vi "Test program 5.vi"() -> ()   [LabVIEW 2013, in "Keithly user program.lvlib"]
uses:
  Keithly user program.lvlib
  Typedefs/KE622x -- On Off Control.ctl
  Configure/Output/Typedefs/KE6221 -- Output Response.ctl
  Configure/Source/Typedefs/KE622x -- Current Range.ctl
  Configure/Source/Typedefs/KE622x -- Current Level.ctl
  Configure/Source/Typedefs/KE622x -- Voltage Limit.ctl
  Configure/Utility/Typedefs/KE622x -- Instrument Type.ctl
panel:
  in  "Current Level (A) 2":T1=0.1 min=-0.105 max=0.105 format="%.4p"
  in  "stop 2":bool
  in  "stop":bool
  out "XY Graph":cluster{"X":dbl, "Y":dbl}[](graph)
  in  "2182 -A Params In":T2={"Auto Range?"=FALSE, "Man / Selected\n       Range"=enum."10mV", "Enable Digital\n       Filter?"=FALSE, "Filter Type"=enum."Movin", "Filter Count"=1, "      Filter\nWindow (%)"=0.01, "Enable Analog\n       Filter?"=FALSE, "NPLCs"=5} {"NPLCs" min=1 max=10; "Filter\nWindow (%)" min=0.01 max=10.0 step=0.01 format="%.2f"; "Filter Count" min=1 max=100}
  in  "Voltage Limit (V)":T3=10.0 min=0.1 max=105.0 step=0.01 format="%.2p"
  in  "Current Level (A)":T1=0.1 min=-0.105 max=0.105 format="%.4p"
  in  "Current Range":T4
  in  "KE6221 Output Response":T5=enum."Slow"
  in  "Analog Filter State":T6
  in  "VISA resource name":refnum<visa-resource-name>
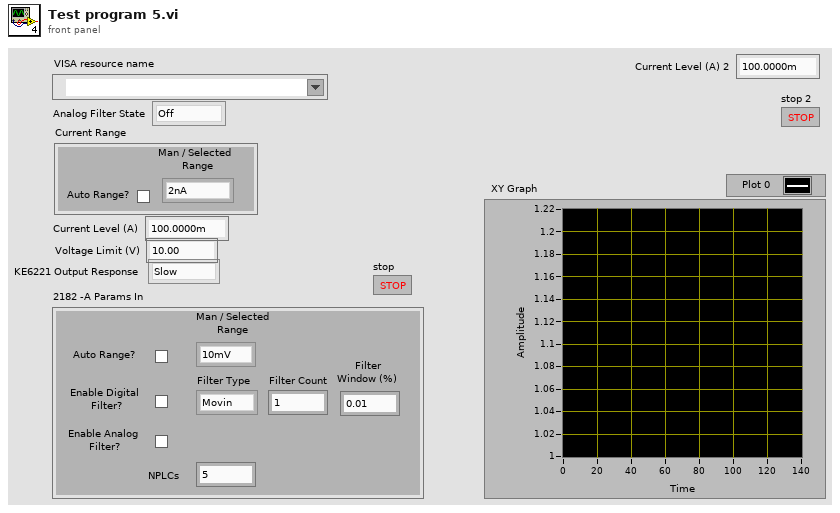
[diagram p1: front panel]
types:
  T1 = typedef "Keithly user program.lvlib/KE622x -- Current Level.ctl" = dbl
  T2 = cluster{"Auto Range?":bool, "Man / Selected\n       Range":enum16{"10mV", "100mV", "1V", "10V", "100V"}, "Enable Digital\n       Filter?":bool, "Filter Type":enum16{"Movin", "Repeat"}, "Filter Count":u32, "      Filter\nWindow (%)":dbl, "Enable Analog\n       Filter?":bool, "NPLCs":u32}
  T3 = typedef "Keithly user program.lvlib/KE622x -- Voltage Limit.ctl" = dbl
  T4 = typedef "Keithly user program.lvlib/KE622x -- Current Range.ctl" = cluster{"Auto Range?":bool, "Man / Selected\n        Range":enum16{"2nA", "20nA", "200nA", "2uA", "20uA", "200uA", "2mA", "20mA", "100mA"}}
  T5 = typedef "Keithly user program.lvlib/KE6221 -- Output Response.ctl" = enum16{"Fast", "Slow"}
  T6 = typedef "Keithly user program.lvlib/KE622x -- On Off Control.ctl" = enum16{"Off", "On"}
  T7 = typedef "Keithly user program.lvlib/KE622x -- Instrument Type.ctl" = enum16{"KE6220", "KE6221"}
  T8 = cluster{"Auto Range?":bool, "Man / Selected\n        Range":u16, "Enable Digital\n       Filter?":bool, "Filter Type":u16, "Filter Count":u32, "      Filter\nWindow (%)":dbl, "Enable Analog\n       Filter?":bool, "NPLCs":u32}
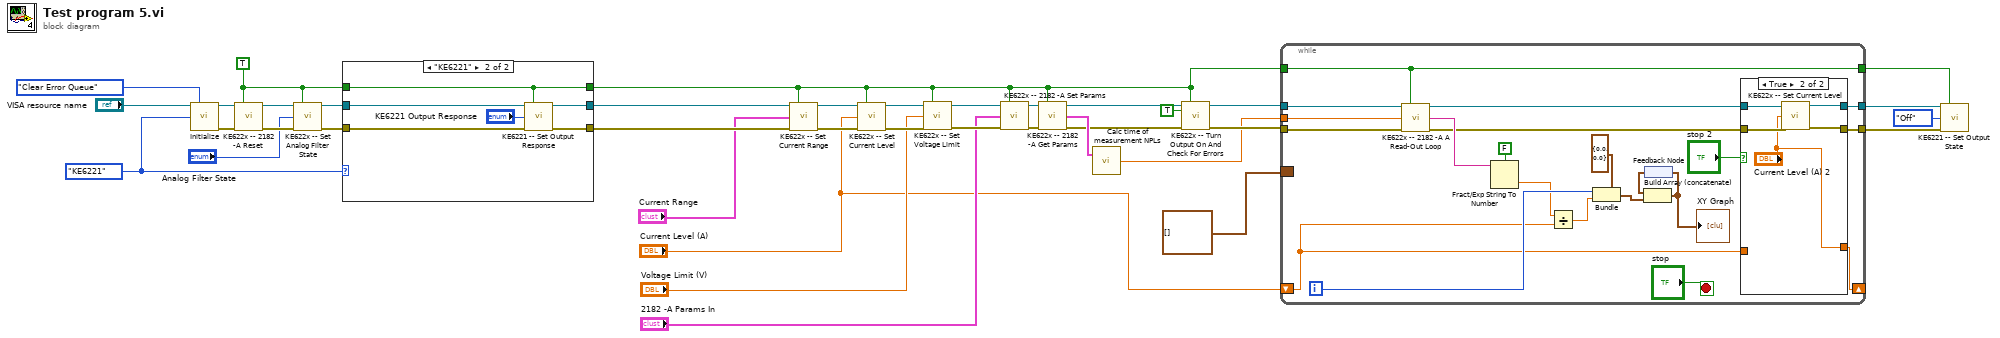
[diagram p0: block diagram]
diagram:
  w28 = TRUE ("Check For SCPI Errors? (T)")
  w29 = KE622x_--_Instrument_Type."KE6221" ("Instrument Type")
  n1 = call "Initialize.vi"("VISA resource name"="VISA resource name", "Error Queue Option"=enum16{"Clear Error Queue", "Error Query"}."Clear Error Queue", "Instrument Type"=w29) -> ("VISA resource name out"=w36:refnum<visa-resource-name>, "error out"=w35:errorcluster)  [unwired: 11 in]
  n2 = call "KE622x -- 2182 -A Reset.vi"("622x Resource In"=w36, "Check For SCPI Errors? (T)"=w28, "error in (no error)"=w35) -> ("622x Resource Out (dupl)"=w34:refnum<visa-resource-name>, "error out"=w33:errorcluster)  [unwired: 11 in]
  n3 = call "KE622x -- Set Analog Filter State.vi"("Resource In"=w34, "Check For SCPI Errors? (T)"=w28, "Analog Filter State"="Analog Filter State", "error in (no error)"=w33) -> ("Resource Out (dupl)"=w31:refnum<visa-resource-name>, "error out"=w30:errorcluster)  [unwired: 10 in]
  n4 = case shown="\"KE6221\"" w29 {
    tunnel: w31 -> [w40 w47]
    tunnel: w30 -> [w39 w46]
    tunnel: [w41 w42] -> w6
    tunnel: w28 -> [w41 w42]
    tunnel: [w40 w44] -> w27
    tunnel: [w39 w43] -> w26
    frame "KE6220", Default {
    }
    frame "KE6221" {
      n5 = call "KE6221 -- Set Output Response.vi"("Resource In"=w47, "Check For SCPI Errors? (T)"=w42, "KE6221 Output Response"="KE6221 Output Response", "error in (no error)"=w46) -> ("Resource Out (dupl)"=w44:refnum<visa-resource-name>, "error out"=w43:errorcluster)  [unwired: 10 in]
    }
  }
  n6 = call "KE622x -- Set Current Range.vi"("Resource In"=w27, "Check For SCPI Errors? (T)"=w6, "Current Range"="Current Range", "error in (no error)"=w26) -> ("Resource Out (dupl)"=w24:refnum<visa-resource-name>, "error out"=w23:errorcluster)  [unwired: 10 in]
  n7 = call "KE622x -- Set Current Level.vi"("Resource In"=w24, "Check For SCPI Errors? (T)"=w6, "Current Level (A)"="Current Level (A)", "error in (no error)"=w23) -> ("Resource Out (dupl)"=w22:refnum<visa-resource-name>, "error out"=w21:errorcluster)  [unwired: 10 in]
  n8 = call "KE622x -- Set Voltage Limit.vi"("Resource In"=w22, "Check For SCPI Errors? (T)"=w6, "Voltage Limit (V)"="Voltage Limit (V)", "error in (no error)"=w21) -> ("Resource Out (dupl)"=w19:refnum<visa-resource-name>, "error out"=w18:errorcluster)  [unwired: 10 in]
  n9 = call "KE622x -- 2182 -A Set Params.vi"("622x Resource In"=w19, "Check For SCPI Errors? (T)"=w6, "2182 -A Params In"="2182 -A Params In", "error in (no error)"=w18) -> ("622x Resource Out (dupl)"=w16:refnum<visa-resource-name>, "error out"=w15:errorcluster)  [unwired: 10 in]
  n10 = call "KE622x -- 2182 -A Get Params.vi"("622x Resource In"=w16, "Check For SCPI Errors? (T)"=w6, "error in (no error)"=w15) -> ("622x Resource Out (dupl)"=w13:refnum<visa-resource-name>, "2182 -A Params"=w14:T8, "error out"=w12:errorcluster)  [unwired: 10 in]
  n11 = call "Calc time of measurement NPLs.vi"("2182 -A Params"=w14) -> ("Time of one measurement"=w7:dbl)  [unwired: 1 in]
  n12 = call "KE622x -- Turn Output On And Check For Errors.vi"("Resource In"=w13, "Check For SCPI Errors? (T)"=w6, "Turn Off Output If Compliance?"=TRUE, "error in (no error)"=w12) -> ("Resource Out (dupl)"=w10:refnum<visa-resource-name>, "error out"=w9:errorcluster)  [unwired: 8 in, 2 out]
  n13 = while {
    tunnel: w10 -> [w68]
    tunnel: w9 -> [w67]
    tunnel: w7 -> [w66]
    border: cluster{"X":dbl, "Y":dbl}[] [] ("XY Graph") -> [_]
    tunnel: [w54] -> w4
    tunnel: [w53] -> w3
    tunnel: w6 -> [w62]
    tunnel: [w62] -> w2
    shift-right: [w48] -> _
    shift-left: "Current Level (A)" -> [w49]
    i -> [w58]
    stop <- "stop" stop-if-true
    n14 = call "KE622x -- 2182 -A A Read-Out Loop.vi"("622x Resource In"=w68, "Check For SCPI Errors? (T)"=w62, "Time of one measurement"=w66, "error in (no error)"=w67) -> ("622x Resource Out (dupl)"=w55:refnum<visa-resource-name>, "2182-A Reponse String"=w65:string, "error out"=w56:errorcluster)  [unwired: 9 in]
    n15 = Fract/Exp String To Number(use system decimal point (T)=FALSE, string=w65) -> (number=w51:dbl)  [unwired: 2 in, 1 out]
    n16 = Divide(x=w51, y=w49) -> (x/y=w50:T1)
    n17 = Bundle(cluster=cluster{"X":dbl, "Y":dbl} {"X"=0.0, "Y"=0.0}, "X"=w58, "Y"=w50) -> (w59:cluster{"X":dbl, "Y":dbl})
    n18 = feedback #1() -> (w60:cluster{"X":dbl, "Y":dbl}[])
    n19 = Build Array (concatenate)(w60, w59) -> (w57:cluster{"X":dbl, "Y":dbl}[])
    "XY Graph" <- w57
    n20 = feedback-in #1(w57) -> ()
    n21 = case shown="True" "stop 2" {
      tunnel: w56 -> [w70 w74]
      tunnel: w55 -> [w71 w76]
      tunnel: [w71 w75] -> w54
      tunnel: [w70 w73] -> w53
      tunnel: w49 -> [w69 _]
      tunnel: [w69 "Current Level (A) 2"] -> w48
      frame False {
      }
      frame True {
        n22 = call "KE622x -- Set Current Level.vi"("Resource In"=w76, "Current Level (A)"="Current Level (A) 2", "error in (no error)"=w74) -> ("Resource Out (dupl)"=w75:refnum<visa-resource-name>, "error out"=w73:errorcluster)  [unwired: 11 in]
      }
    }
  }
  n23 = call "KE6221 -- Set Output State.vi"("Resource In"=w4, "Check For SCPI Errors? (T)"=w2, "Output State"=KE622x_--_On_Off_Control."Off", "error in (no error)"=w3) -> ()  [unwired: 10 in, 2 out]
